vi "Temperatura.vi"() -> ()   [LabVIEW 2017, in "GUI.lvlib"]
uses:
  Libraries/GUI/GUI.lvlib
  Libraries/Akwizycja/GUI Control.ctl
  Libraries/Akwizycja/Data Enum.ctl
  <vilib>/Delacor/Delacor QMH/Libraries/Message Queue_class/Delacor_lib_QMH_Enqueue Message (Single).vi
  <vilib>/Delacor/Delacor QMH/Libraries/Message Queue_class/Delacor_lib_QMH_Message Queue.lvclass
panel:
  out "Slave 6":T1
  out "Slave 5":T2
  out "Slave 4":T3
  out "Slave 3":T4
  out "Slave 2":T5
  out "STM":T6
  in  "Automatyczne przełączanie":bool
  in  "Czas przełączania":dbl=15.0 min=15.0 max=600.0 step=1.0
  in  "Podgląd":T7
  out "Fuel Flows":dbl[][](array[numeric])
  in  "f_q":dbl[][](array[numeric])
  out "Temperatures":dbl[][](array[numeric])
  in  "Array 4":dbl[][](array[numeric])
  in  "Stop":bool
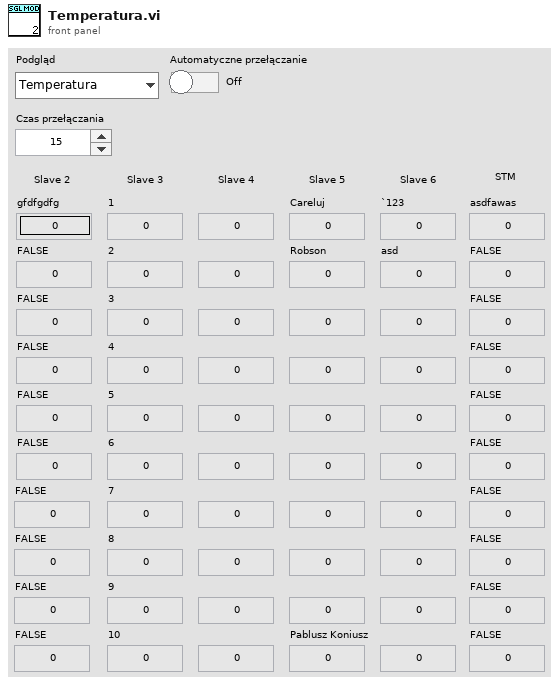
[diagram p1: front panel]
types:
  T1 = cluster{"Zmienna 51":dbl, "Zmienna 52":dbl, "Zmienna 53":dbl, "Zmienna 54":dbl, "Zmienna 55":dbl, "Zmienna 56":dbl, "Zmienna 57":dbl, "Zmienna 58":dbl, "Zmienna 59":dbl, "Zmienna 60":dbl}
  T2 = cluster{"Zmienna 41":dbl, "Zmienna 42":dbl, "Zmienna 43":dbl, "Zmienna 44":dbl, "Zmienna 45":dbl, "Zmienna 46":dbl, "Zmienna 47":dbl, "Zmienna 48":dbl, "Zmienna 49":dbl, "Zmienna 50":dbl}
  T3 = cluster{"Zmienna 31":dbl, "Zmienna 32":dbl, "Zmienna 33":dbl, "Zmienna 34":dbl, "Zmienna 35":dbl, "Zmienna 36":dbl, "Zmienna 37":dbl, "Zmienna 38":dbl, "Zmienna 39":dbl, "Zmienna 40":dbl}
  T4 = cluster{"Zmienna 21":dbl, "Zmienna 22":dbl, "Zmienna 23":dbl, "Zmienna 24":dbl, "Zmienna 25":dbl, "Zmienna 26":dbl, "Zmienna 27":dbl, "Zmienna 28":dbl, "Zmienna 29":dbl, "Zmienna 30":dbl}
  T5 = cluster{"Zmienna 11":dbl, "Zmienna 12":dbl, "Zmienna 13":dbl, "Zmienna 14":dbl, "Zmienna 15":dbl, "Zmienna 16":dbl, "Zmienna 17":dbl, "Zmienna 18":dbl, "Zmienna 19":dbl, "Zmienna 20":dbl}
  T6 = cluster{"Zmienna 1":dbl, "Zmienna 2":dbl, "Zmienna 3":dbl, "Zmienna 4":dbl, "Zmienna 5":dbl, "Zmienna 6":dbl, "Zmienna 7":dbl, "Zmienna 8":dbl, "Zmienna 9":dbl, "Zmienna 10":dbl}
  T7 = typedef "GUI Control.ctl" = enum16{"Temperatura", "Przepływ"}
  T8 = typedef "Data Enum.ctl" = enum16{"get_data", "get_data_switch"}
  T9 = cluster{"Controls[]":refnum<vi>[], "Controls[]":refnum<vi>[], "Controls[]":refnum<vi>[], "Controls[]":refnum<vi>[], "Controls[]":refnum<vi>[], "Controls[]":refnum<vi>[]}
  T10 = cluster{"Temperatures[0]":dbl, "Temperatures[1]":dbl, "Temperatures[2]":dbl, "Temperatures[3]":dbl, "Temperatures[4]":dbl, "Temperatures[5]":dbl, "Temperatures[6]":dbl, "Temperatures[7]":dbl, "Temperatures[8]":dbl, "Temperatures[9]":dbl}
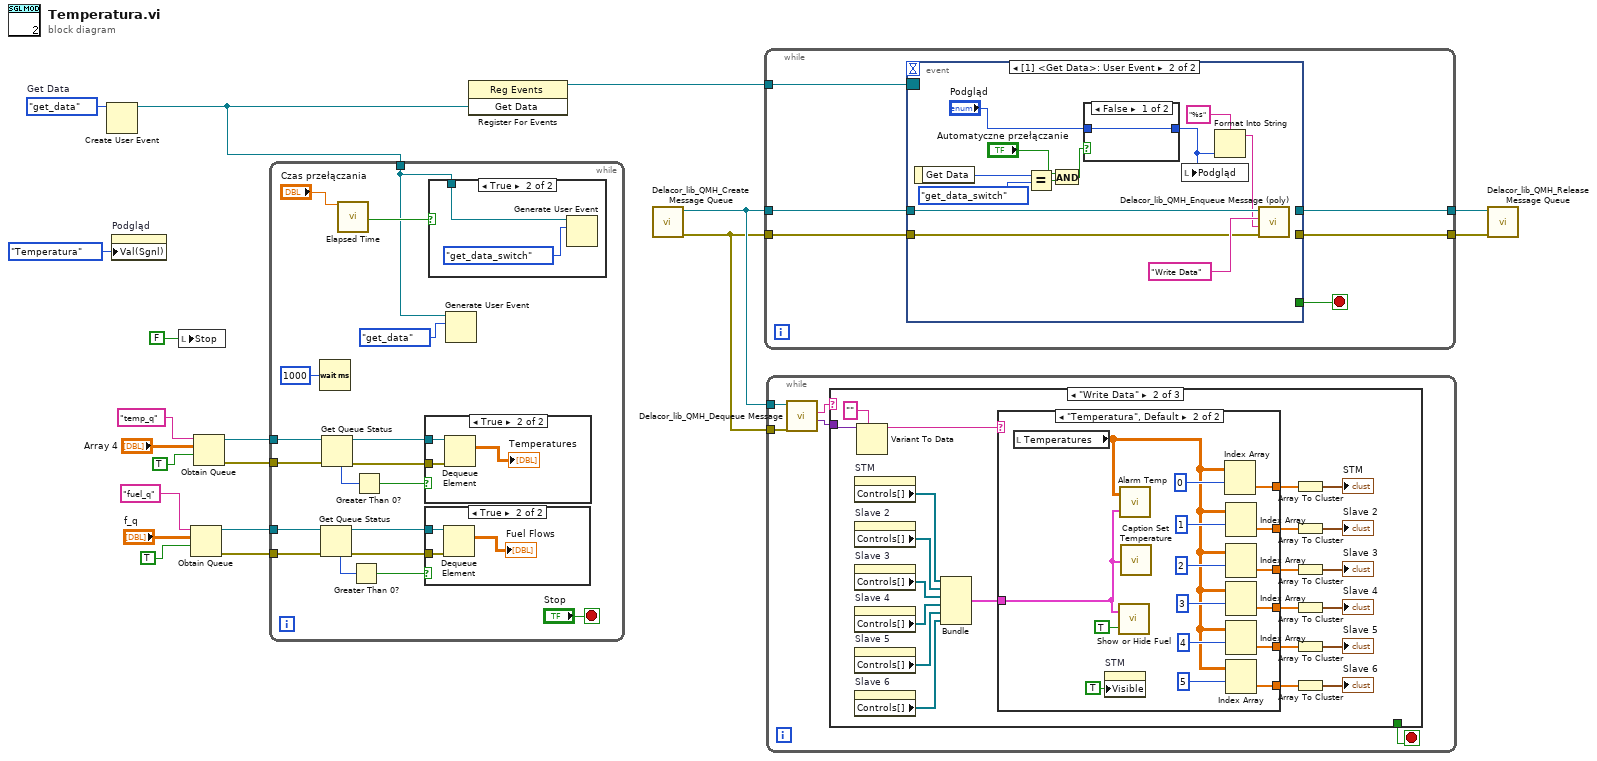
[diagram p0: block diagram]
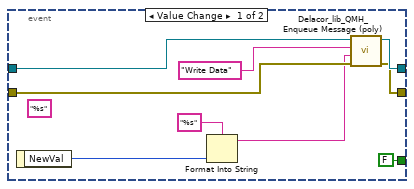
[diagram p5: hidden frame]
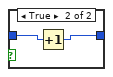
[diagram p6: hidden frame]
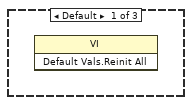
[diagram p7: hidden frame]
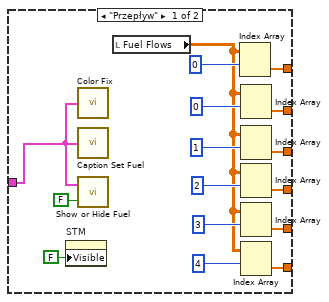
[diagram p8: hidden frame]
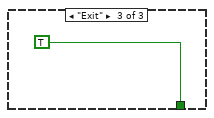
[diagram p9: hidden frame]
diagram:
  w7 = Data_Enum."get_data"  # Get Data
  n1 = Create User Event(user event datatype=w7) -> (user event=w2:refnum<user-event>)  [unwired: 1 in, 1 out]
  n2 = property on="Podgląd" class="Enum (strict)"("Val(Sgnl)"=GUI_Control."Temperatura" ("Value (Signaling)")) -> ()  [unwired: 2 in, 2 out]
  n3 = local write "Stop"(FALSE) -> ()
  n4 = Obtain Queue(name (unnamed)="fuel_q", element data type="f_q", create if not found? (T)=TRUE) -> (queue out=w9:refnum<queue>, error out=w8:errorcluster)  [unwired: 2 in, 1 out]
  n5 = Obtain Queue(name (unnamed)="temp_q", element data type="Array 4", create if not found? (T)=TRUE) -> (queue out=w14:refnum<queue>, error out=w13:errorcluster)  [unwired: 2 in, 1 out]
  n6 = while {
    tunnel: w14 -> [w33]
    tunnel: w13 -> [w32]
    tunnel: w9 -> [w26]
    tunnel: w8 -> [w27]
    tunnel: w2 -> [w21]
    stop <- "Stop" stop-if-true
    n7 = Wait (ms)(milliseconds to wait=u32 1000) -> ()  [unwired: 1 out]
    n8 = Get Queue Status(queue=w26, error in (no error)=w27) -> (queue out=w22:refnum<queue>, error out=w23:errorcluster, # elements in queue=w25:i32)  [unwired: 1 in, 5 out]
    n9 = Get Queue Status(queue=w33, error in (no error)=w32) -> (queue out=w29:refnum<queue>, error out=w30:errorcluster, # elements in queue=w31:i32)  [unwired: 1 in, 5 out]
    n10 = call "Elapsed Time"("Time Target (s)"="Czas przełączania") -> ("Time has Elapsed"=w36:bool)  [unwired: 11 in, 7 out]
    n11 = Greater Than 0?(x=w25) -> (x > 0?=w24:bool)
    n12 = Greater Than 0?(x=w31) -> (x > 0?=w28:bool)
    n13 = case shown="True" w28 {
      tunnel: w30 -> [_ w42]
      tunnel: w29 -> [_ w41]
      frame False {
      }
      frame True {
        n14 = Dequeue Element(queue=w41, error in (no error)=w42) -> (element=→"Temperatures":dbl[][])  [unwired: 1 in, 3 out]
      }
    }
    n15 = case shown="True" w24 {
      tunnel: w22 -> [_ w40]
      tunnel: w23 -> [_ w39]
      frame False {
      }
      frame True {
        n16 = Dequeue Element(queue=w40, error in (no error)=w39) -> (element=→"Fuel Flows":dbl[][])  [unwired: 1 in, 3 out]
      }
    }
    n17 = case shown="True" w36 {
      tunnel: w21 -> [_ w45]
      frame False {
      }
      frame True {
        n18 = Generate User Event(user event=w45, event data cluster=Data_Enum."get_data_switch") -> ()  [unwired: 2 in, 2 out]
      }
    }
    n19 = Generate User Event(user event=w21, event data cluster=Data_Enum."get_data" ("event data")) -> ()  [unwired: 2 in, 2 out]
  }
  n20 = register-events(w2) -> (reference out=w19:refnum<event-registration>)  [unwired: 2 in, 1 out]
  n21 = call <vilib>:"Delacor_lib_QMH_Create Message Queue.vi"() -> ("error out"=w5:errorcluster, "Message Queue"=w6:refnum<class "Delacor_lib_QMH_Message Queue.lvclass">)  [unwired: 10 in]
  n22 = while {
    tunnel: w6 -> [w51]
    tunnel: w5 -> [w50]
    tunnel: [w49] -> w4
    tunnel: [w48] -> w3
    tunnel: w19 -> [w46]
    stop <- w47 stop-if-true
    n23 = event shown="[1] <Get Data>: User Event" {
      selector: w46 -> [_ _]
      dyn-events: _ -> [_ _]
      timeout: _ -> [_ _]
      tunnel: w51 -> [w59 w70]
      tunnel: w50 -> [w58 w71]
      tunnel: [w57 _] -> w49
      tunnel: [w56 _] -> w48
      tunnel: [FALSE _] -> w47
      event Value Change {
        (unwired) "%s" ("format string")
        n24 = event-data() -> ("NewVal"=w54:T7)  [unwired: 1 in]
        n25 = Format Into String(format string="%s", w54) -> (resulting string=w53:string)  [unwired: 2 in, 1 out]
        n26 = call-poly <vilib>:"Delacor_lib_QMH_Enqueue Message (poly).vi"("error in (no error)"=w58, "Message Data"=w53, "Message"="Write Data", "Message Queue in"=w59) -> ("error out"=w56:errorcluster, "Message Queue out"=w57:refnum<class "Delacor_lib_QMH_Message Queue.lvclass">)  [unwired: 6 in]
      }
      event User Event {
        n27 = event-data() -> ("Get Data"=w67:T8)  [unwired: 1 in]
        n28 = Equal?(x=w67, y=Data_Enum."get_data_switch") -> (x = y?=w65:bool)
        n29 = And(x="Automatyczne przełączanie", y=w65) -> (x .and. y?=w63:bool)
        n30 = case shown="False" w63 {
          tunnel: [w73 w75] -> w61
          tunnel: "Podgląd" -> [w73 w74]
          frame False {
          }
          frame True {
            n31 = Increment(x=w74) -> (x+1=w75:T7)
          }
        }
        n32 = local write "Podgląd"(w61) -> ()
        n33 = Format Into String(format string="%s", w61) -> (resulting string=w68:string)  [unwired: 2 in, 1 out]
        n34 = call-poly <vilib>:"Delacor_lib_QMH_Enqueue Message (poly).vi"("error in (no error)"=w71, "Message Data"=w68, "Message"="Write Data", "Message Queue in"=w70) -> ()  [unwired: 6 in, 2 out]
      }
    }
  }
  n35 = while {
    tunnel: w6 -> [w80]
    tunnel: w5 -> [w79]
    stop <- w76 stop-if-true
    n36 = call-dynamic "Delacor_lib_QMH_Dequeue Message.vi"("error in (no error)"=w79, "Message Queue in"=w80) -> ("Message Data"=w78:variant, "Message"=w77:string)  [unwired: 6 in, 2 out]
    n37 = case shown="\"Write Data\"" w77 {
      tunnel: w78 -> [_ w96 _]
      tunnel: [_ _ TRUE] -> w76
      frame Default {
        n38 = invoke class="VI" method="Default Vals.Reinit All"() -> ()  [unwired: 3 in, 3 out]
      }
      frame "Write Data" {
        n39 = property on="STM" class="Clust (strict)"() -> ("Controls[]"=w87:refnum<vi>[])  [unwired: 2 in, 2 out]
        n40 = property on="Slave 2" class="Clust (strict)"() -> ("Controls[]"=w86:refnum<vi>[])  [unwired: 2 in, 2 out]
        n41 = property on="Slave 3" class="Clust (strict)"() -> ("Controls[]"=w85:refnum<vi>[])  [unwired: 2 in, 2 out]
        n42 = property on="Slave 4" class="Clust (strict)"() -> ("Controls[]"=w83:refnum<vi>[])  [unwired: 2 in, 2 out]
        n43 = property on="Slave 5" class="Clust (strict)"() -> ("Controls[]"=w84:refnum<vi>[])  [unwired: 2 in, 2 out]
        n44 = property on="Slave 6" class="Clust (strict)"() -> ("Controls[]"=w82:refnum<vi>[])  [unwired: 2 in, 2 out]
        n45 = Variant To Data(type="", Variant=w96) -> (data=w94:string)  [unwired: 1 in, 1 out]
        n46 = Bundle("Controls[]"=w87, "Controls[]"=w86, "Controls[]"=w85, "Controls[]"=w83, "Controls[]"=w84, "Controls[]"=w82) -> (w81:T9)  [unwired: 1 in]
        n47 = case shown="\"Temperatura\", Default" w94 {
          tunnel: [w110 w128] -> w93
          tunnel: [w109 w127] -> w92
          tunnel: [w108 w126] -> w91
          tunnel: [w107 w125] -> w90
          tunnel: [w106 w124] -> w89
          tunnel: [w105 w123] -> w88
          tunnel: w81 -> [w103 w119]
          frame "Przepływ" {
            n48 = property on="STM" class="Clust (strict)"("Visible"=FALSE) -> ()  [unwired: 2 in, 2 out]
            n49 = call "Color Fix.vi"("Reference Cluster"=w103) -> ()
            n50 = call "Caption Set Fuel.vi"("Reference Cluster"=w103) -> ()
            n51 = call "Show or Hide Fuel.vi"("Bool"=FALSE, "Reference Cluster"=w103) -> ()
            n52 = local read "Fuel Flows"() -> (w112:dbl[][])
            n53 = Index Array(array=w112, index (row)=0) -> (element=w110:dbl[])  [unwired: 1 in]
            n54 = Index Array(array=w112, index (row)=0) -> (element=w109:dbl[])  [unwired: 1 in]
            n55 = Index Array(array=w112, index (row)=1) -> (element=w108:dbl[])  [unwired: 1 in]
            n56 = Index Array(array=w112, index (row)=2) -> (element=w107:dbl[])  [unwired: 1 in]
            n57 = Index Array(array=w112, index (row)=3) -> (element=w106:dbl[])  [unwired: 1 in]
            n58 = Index Array(array=w112, index (row)=4) -> (element=w105:dbl[])  [unwired: 1 in]
          }
          frame "Temperatura", Default {
            n59 = local read "Temperatures"() -> (w120:dbl[][])
            n60 = property on="STM" class="Clust (strict)"("Visible"=TRUE) -> ()  [unwired: 2 in, 2 out]
            n61 = call "Show or Hide Fuel.vi"("Bool"=TRUE, "Reference Cluster"=w119) -> ()
            n62 = call "Alarm Temp.vi"("Reference Cluster"=w119, "Temperatures"=w120) -> ()
            n63 = call "Caption Set Temperature.vi"("Reference Cluster"=w119) -> ()
            n64 = Index Array(array=w120, index (row)=0) -> (element=w128:dbl[])  [unwired: 1 in]
            n65 = Index Array(array=w120, index (row)=1) -> (element=w127:dbl[])  [unwired: 1 in]
            n66 = Index Array(array=w120, index (row)=2) -> (element=w126:dbl[])  [unwired: 1 in]
            n67 = Index Array(array=w120, index (row)=3) -> (element=w125:dbl[])  [unwired: 1 in]
            n68 = Index Array(array=w120, index (row)=4) -> (element=w124:dbl[])  [unwired: 1 in]
            n69 = Index Array(array=w120, index (row)=5) -> (element=w123:dbl[])  [unwired: 1 in]
          }
        }
        n70 = Array To Cluster(array=w93) -> (cluster=→"STM":T10)
        n71 = Array To Cluster(array=w92) -> (cluster=→"Slave 2":T10)
        n72 = Array To Cluster(array=w91) -> (cluster=→"Slave 3":T10)
        n73 = Array To Cluster(array=w90) -> (cluster=→"Slave 4":T10)
        n74 = Array To Cluster(array=w89) -> (cluster=→"Slave 5":T10)
        n75 = Array To Cluster(array=w88) -> (cluster=→"Slave 6":T10)
      }
      frame "Exit" {
      }
    }
  }
  n76 = call-dynamic "Delacor_lib_QMH_Release Message Queue.vi"("error in (no error)"=w3, "Message Queue"=w4) -> ()  [unwired: 9 in, 1 out]
